vi "Defer Panel Updates_csm.vi"(8 "Error In":errorcluster, 10 "Defer Updates?":bool, 11 "VI Reference (Caller)":refnum<vi>) -> (0 "Error Out":errorcluster, 3 "VI Reference (Caller) 2":refnum<vi>)   [LabVIEW 2017, in "csm-tool-support.lvlib"]
doc: "Defers or Restores Panel Updates for the specified VI.\nThis VI tracks the number of times a defer/restore is made for each VI so that multiple defers must be matched with multiple restores. A Defer or Restore will be attempted even if an error exists on input.\n\nAuthored by Shawn Walpole\nsupport@mooregoodideas.com\nwww.mooregoodideas.com\n\nCopyright (c) 2010, Moore Good Ideas, Inc.\n\nAll rights reserved.\n\nRedistribution and use in source and binary forms, with or without modification, are permitted provided that the following conditions are met:\n\n * Redistributions of source code must retain the above copyright notice, this list of conditions and the following disclaimer.\n * Redistributions in binary form must reproduce the above copyright notice, this list of conditions and the following disclaimer in the documentation and/or other materials provided with the distribution.\n * Neither the name of Moore Good Ideas, Inc. nor the names of its contributors may be used to endorse or promote products derived from this software without specific prior written permission.\n\nTHIS SOFTWARE IS PROVIDED BY THE COPYRIGHT HOLDERS AND CONTRIBUTORS \"AS IS\" AND ANY EXPRESS OR IMPLIED WARRANTIES, INCLUDING, BUT NOT LIMITED TO, THE IMPLIED WARRANTIES OF MERCHANTABILITY AND FITNESS FOR A PARTICULAR PURPOSE ARE DISCLAIMED. IN NO EVENT SHALL THE COPYRIGHT OWNER OR CONTRIBUTORS BE LIABLE FOR ANY DIRECT, INDIRECT, INCIDENTAL, SPECIAL, EXEMPLARY, OR CONSEQUENTIAL DAMAGES (INCLUDING, BUT NOT LIMITED TO, PROCUREMENT OF SUBSTITUTE GOODS OR SERVICES; LOSS OF USE, DATA, OR PROFITS; OR BUSINESS INTERRUPTION) HOWEVER CAUSED AND ON ANY THEORY OF LIABILITY, WHETHER IN CONTRACT, STRICT LIABILITY, OR TORT (INCLUDING NEGLIGENCE OR OTHERWISE) ARISING IN ANY WAY OUT OF THE USE OF THIS SOFTWARE, EVEN IF ADVISED OF THE POSSIBILITY OF SUCH DAMAGE."
uses:
  csm-tool-support.lvlib
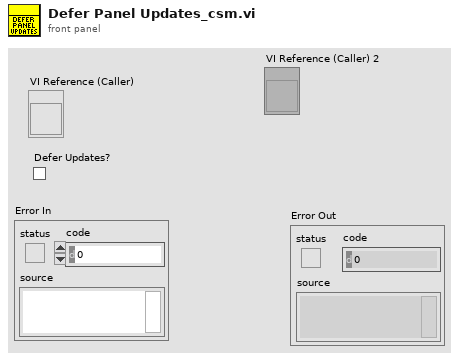
[diagram p1: front panel]
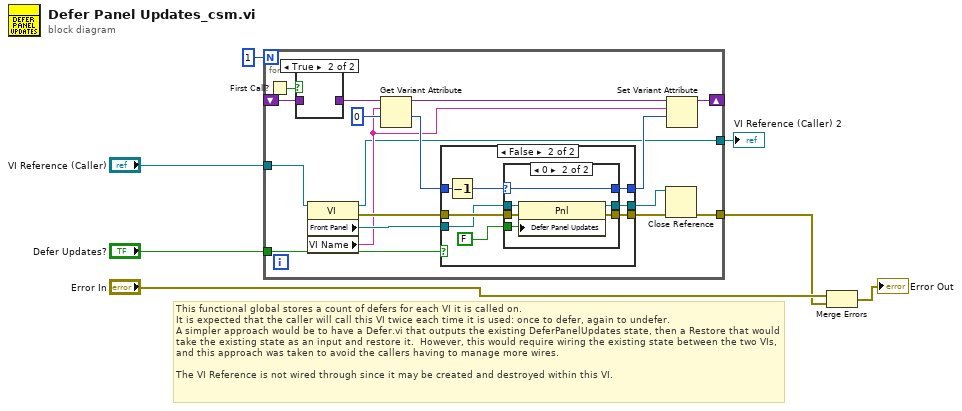
[diagram p0: block diagram]
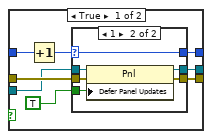
[diagram p3: hidden frame]
diagram:
  # "This functional global stores a count of defers for each VI it is called on.\nIt is expected that the caller will call this VI twice each time it is used: once to defer, again to undefer.\nA simpler approach would be to have a Defer.vi that outputs the existing DeferPanelUpdates state, then a Restore that would take the existing state as an input and restore it.  However, this would require wiring the existing state between the two VIs, and this approach was taken to avoid the callers having to manage more wires.\n\nThe VI Reference is not wired through since it may be created and destroyed within this VI."
  n1 = for {
    N: 1 -> [_]
    shift-right: [w24] -> _
    shift-left: _ -> [w16]
    tunnel: "VI Reference (Caller)" -> [w9]
    tunnel: "Defer Updates?" -> [w20]
    tunnel: [w8] -> w1
    tunnel: [w10] -> w3
    n2 = First Call?() -> (First Call?: T/F=w17:bool)
    n3 = case shown="True" w17 {
      tunnel: w16 -> [w25 _]
      tunnel: [w25 _] -> w15
      frame False {
      }
      frame True {
      }
    }
    n4 = property class="VI"(reference=w9) -> (reference out=w8:refnum<vi>, error out=w21:errorcluster, "Front Panel"=w18:refnum<vi>, "VI Name"=w13:string)  [unwired: 1 in]
    n5 = Get Variant Attribute(Variant=w15, name=w13, default value (empty Variant)=0) -> (duplicate Variant=w23:variant, value=w19:i32)  [unwired: 1 in, 2 out]
    n6 = case shown="False" w20 {
      tunnel: w21 -> [w33 w50]
      tunnel: w19 -> [w28 w45]
      tunnel: w18 -> [w32 w49]
      tunnel: [w31 w48] -> w12
      tunnel: [w26 w43] -> w14
      tunnel: [w29 w46] -> w11
      frame True {
        n7 = Increment(x=w28) -> (x+1=w27:i32)
        n8 = case shown="1" w27 {
          selector: w27 -> [w34 w37]
          tunnel: w33 -> [w36 w42]
          tunnel: w32 -> [w35 w41]
          tunnel: TRUE -> [_ w40]
          tunnel: [w36 w39] -> w31
          tunnel: [w35 w38] -> w29
          tunnel: [w34 w37] -> w26
          frame Default {
          }
          frame 1 {
            n9 = property class="Pnl"(reference=w41, error in=w42, "Defer Panel Updates"=w40) -> (reference out=w38:refnum<vi>, error out=w39:errorcluster)
          }
        }
      }
      frame False {
        n10 = Decrement(x=w45) -> (x-1=w44:i32)
        n11 = case shown="0" w44 {
          selector: w44 -> [w51 w54]
          tunnel: w50 -> [w53 w59]
          tunnel: w49 -> [w52 w58]
          tunnel: FALSE -> [_ w57]
          tunnel: [w53 w56] -> w48
          tunnel: [w52 w55] -> w46
          tunnel: [w51 w54] -> w43
          frame Default {
          }
          frame 0 {
            n12 = property class="Pnl"(reference=w58, error in=w59, "Defer Panel Updates"=w57) -> (reference out=w55:refnum<vi>, error out=w56:errorcluster)
          }
        }
      }
    }
    n13 = Close Reference(reference=w11, error in (no error)=w12) -> (error out=w10:errorcluster)
    n14 = Set Variant Attribute(Variant=w23, name=w13, value=w14) -> (Variant out=w24:variant)  [unwired: 1 in, 2 out]
  }
  "VI Reference (Caller) 2" <- w1
  n15 = Merge Errors("Error In", w3) -> (→"Error Out":errorcluster)
